vi "CH_LM Event Queue Monitor.vi"() -> ()   [LabVIEW 2012, in "CH_LM.lvlib"]
doc: "This VI is a simple tool to monitor LabMax event queues."
uses:
  CH_LM.lvlib
  CH_LM Event Cluster.ctl
panel:
  out "maximum elements":i32
  in  "intervall / ms":u32=100
  in  "Serial Number":string
  in  "Queue Type":u16(ring) items=["Event Data", "Return Data", "Streaming Data"]
  in  "stop":bool
  out "# pending remove":i32
  out "# pending insert":i32
  out "# elements in queue":i32
  in  "CH_LM Event Cluster":T1
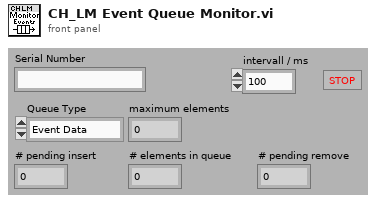
[diagram p1: front panel]
types:
  T1 = typedef "CH_LM.lvlib/CH_LM Event Cluster.ctl" = cluster{"Event Name":string, "Meter Index":i32, "Serial  Number":string, "Data":string, "iStreamingPacket":variant}
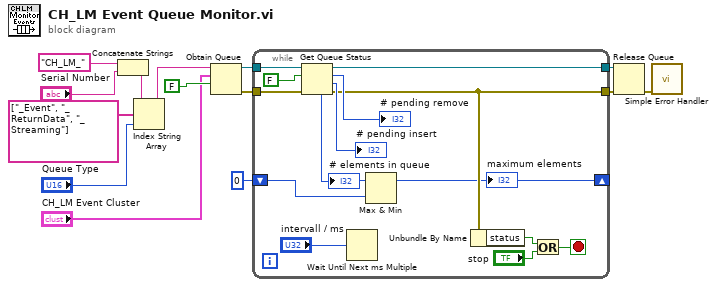
[diagram p0: block diagram]
diagram:
  n1 = Concatenate Strings("CH_LM_", "Serial Number") -> (w9:string)
  n2 = Index String Array(1:"Queue Type", 2:string[] ["_Event", "_ReturnData", "_Streaming"] ("string array"), 3:w9) -> (0:w8:string)
  n3 = Obtain Queue(name (unnamed)=w8, element data type="CH_LM Event Cluster", create if not found? (T)=FALSE) -> (queue out=w14:refnum<queue>, error out=w13:errorcluster)  [unwired: 2 in, 1 out]
  n4 = while {
    tunnel: w14 -> [w28]
    tunnel: w13 -> [w27]
    tunnel: [w20] -> w4
    tunnel: [w19] -> w3
    shift-right: [w15] -> _
    shift-left: 0 -> [w17]
    stop <- w21 stop-if-true
    n5 = Get Queue Status(queue=w28, return elements? (F)=FALSE, error in (no error)=w27) -> (queue out=w19:refnum<queue>, # pending remove=→"# pending remove":i32, # pending insert=→"# pending insert":i32, error out=w20:errorcluster, # elements in queue=w16:i32)  [unwired: 3 out]
    "# elements in queue" <- w16
    n6 = Wait Until Next ms Multiple(millisecond multiple="intervall / ms") -> ()  [unwired: 1 out]
    n7 = Max & Min(x=w16, y=w17) -> (max(x,y)=w15:i32)  [unwired: 1 out]
    "maximum elements" <- w15
    n8 = Unbundle By Name(w20) -> ("status"=w23:bool)
    n9 = Or(x=w23, y="stop") -> (x .or. y?=w21:bool)
  }
  n10 = Release Queue(queue=w3, error in (no error)=w4) -> (error out=w5:errorcluster)  [unwired: 3 out]
  n11 = call <vilib>:"Simple Error Handler.vi"("error in (no error)"=w5) -> ()  [unwired: 1 in, 8 out]
